vi "OAT Get Gap Reference (1 Channel).vi"(0 "scaled signal [EU]":waveform(dbl)={"t0"=timestamp(0 s since 1904-01-01), "dt"=0.0, "Y"=[]}, 2 "reset? (F)":bool, 7 "averaging type":enum16{"Linear", "Exponential"}(ring), 9 "window":T1(ring), 11 "error in (no error)":errorcluster) -> (4 "gap reference [V]":dbl, 15 "error out":errorcluster)   [LabVIEW 2017, in "SoundVib_RefDataProcess.lvlib"]
doc: "Computes the gap reference of the scaled signal you acquire from a DC-coupled displacement transducer channel. You can subtract the gap reference value from a signal to calculate the actual movement that the displacement transducer measures. Wire data to the <B>scaled signal [EU]</B> input to determine the polymorphic instance to use or manually select the instance."
uses:
  <vilib>/addons/Sound and Vibration/Order Analysis/Referece Data Processing/SoundVib_RefDataProcess.lvlib
  <vilib>/addons/_NISVFA/_Shared subVIs/Common/svc_Check for Waveform Parameter Continuity (no state).vi
  <vilib>/measure/madcrms.llb/Basic Averaged DC-RMS for 1 Chan.vi
  <vilib>/addons/_NISVFA/_Shared subVIs/Common/svc_Engineering Units to Unit Label.vi
  <vilib>/addons/_NISVFA/_Shared subVIs/Common/svc_Unit Label to Engineering Units.vi
  <vilib>/measure/NI_MAPro.lvlib
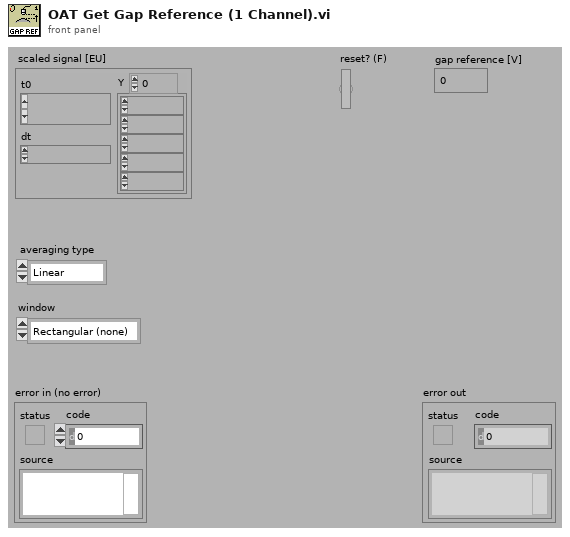
[diagram p1: front panel]
types:
  T1 = enum16{"Rectangular (none)", "Hanning", "Low side lobe"}
  T2 = cluster{"dt":bool, "t0 continuity":bool, "array length":bool, "channel info":bool, "name":bool}
  T3 = typedef "svc_Channel Info.ctl" = cluster{"sensor sensitivity":dbl, "engineering units":T4, "dB reference":dbl, "custom label":string, "weighting filter":T5, "pregain":dbl}
  T4 = typedef "svc_Engineering Units Text Ring.ctl" = u16
  T5 = typedef "svc_Weighting Filter Text Ring.ctl" = u16
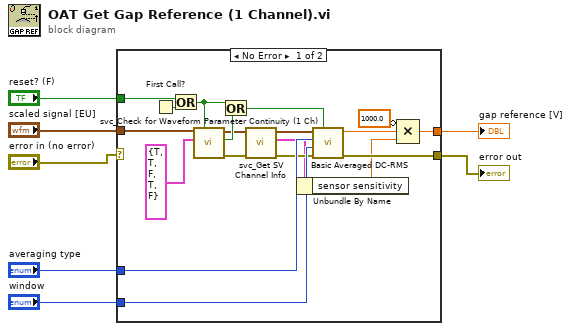
[diagram p0: block diagram]
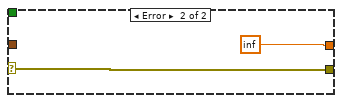
[diagram p2: hidden frame]
diagram:
  n1 = case shown="No Error" "error in (no error)" {
    selector: "error in (no error)" -> [_ w28]
    tunnel: [w23 w28] -> w6
    tunnel: "scaled signal [EU]" -> [w21 _]
    tunnel: "averaging type" -> [w26 _]
    tunnel: "window" -> [w25 _]
    tunnel: "reset? (F)" -> [w22 _]
    tunnel: [w24 inf ("DC value")] -> w1
    frame No Error {
      n2 = First Call?() -> (First Call?: T/F=w20:bool)
      n3 = Or(x=w22, y=w20) -> (x .or. y?=w18:bool)
      n4 = call <vilib>:"svc_Check for Waveform Parameter Continuity (1 Ch).vi"("restart averaging (F)"=w18, "checks for channel parameter change"=T2 {"dt"=TRUE, "t0 continuity"=TRUE, "array length"=FALSE, "channel info"=TRUE, "name"=FALSE}, "scaled signal [EU]"=w21) -> ("error out"=w14:errorcluster, "waveform parameter changed"=w17:bool, "dup scaled signal [EU]"=w15:waveform(dbl))  [unwired: 3 in, 3 out]
      n5 = Or(x=w18, y=w17) -> (x .or. y?=w16:bool)
      n6 = call <vilib>:"svc_Get SV Channel Info.vi"("error in (no error)"=w14, "scaled signal [EU]"=w15) -> ("error out"=w12:errorcluster, "channel info"=w10:T3, "dup scaled signal [EU]"=w13:waveform(dbl))  [unwired: 4 in, 3 out]
      n7 = Unbundle By Name(w10) -> ("sensor sensitivity"=w8:dbl)
      n8 = call-poly <vilib>:"Basic Averaged DC-RMS.vi"("reset"=w16, "error in (no error)"=w12, "window"=w25, "averaging type"=w26, "signal in"=w13) -> ("error out"=w23:errorcluster, "DC value"=w11:dbl)  [unwired: 3 in, 2 out]
      n9 = Compound Arithmetic op=MULTIPLY(invert 1000.0 ("value"), w11, w8) -> (w24:dbl)
    }
    frame Error {
    }
  }
  "error out" <- w6
  "gap reference [V]" <- w1
